vi "Deterministic Errors.Set Error Status.vi"(10 "status (T)":bool=TRUE, 11 "error in":errorcluster) -> (3 "error out":errorcluster)   [LabVIEW 2016, in "Deterministic Error Builder.lvlib"]
uses:
  Deterministic Error Builder.lvlib
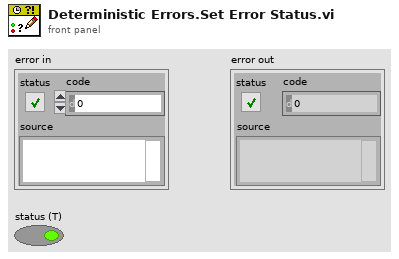
[diagram p1: front panel]
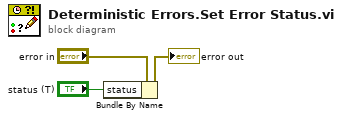
[diagram p0: block diagram]
diagram:
  n1 = Bundle By Name(cluster="error in", "status"="status (T)") -> (→"error out":errorcluster)
